vi "YKMW100 VF0 Relay Status.vi"(0 "VISA session":refnum<visa-resource-name>="MW100", 2 "Semiphore":T1, 5 "Channel_Enum":T2=1 items=["4-20_OUT", "Pres_HI1", "Pres_HI2", "Pres_LOW", "Pres_PIN", "HEATER_TOP", "HEATER_BOT", "T_Shell", "FLOWMETER", "WATT_SENSE", "WH_TICK", "Tc_1", "Tc_2", "Tc_3", "Tc_4", "Tc_5", "Tc_6", "Tc_down", "T_Shell_2", "T_Shell_3", "T_Shell_4", "RTD_IN", "RTD_OUT", "RTD_AMB", "INTF_TEMPFLO", "INTF_READY", "INTF_START", "INTF_STOP", "DRM_LOW", "DRM_HIGH", "PWR_MAIN", "VLV_DUMP", "VLV_OUT", "VLV_IN", "WATT_HOURS", "FLOW(SAMPLE)", "GALLONS", "FLOW(GPM)", "FLOW_CALC_GAIN", "FLOW_CALC_OFFSET", "FLOW_CALC_THRESHOLD", "VLV_DUMP_2", "VLV_OUT_2", "VLV_IN_2", "VLV_DUMP_3", "VLV_OUT_3", "VLV_IN_3", "VLV_DUMP_4", "VLV_OUT_4", "VLV_IN_4", "CHAN_34", "CHAN_35", "CHAN_36"], 9 "Timeout (25000)":u32=1000, 11 "error in (no error)":errorcluster) -> (4 "dup VISA session":refnum<visa-resource-name>, 6 "Output On":bool, 8 "DO Card in Slot 5":bool, 15 "error out":errorcluster)   [LabVIEW 2009]
doc: "This VI sends the message. Then it returns the response."
uses:
  ChannelSettings.ctl
panel:
  out "element":string
  out "Numeric":i32
  out "Local?":bool
  out "Read Array":string[](array[string])
  out "ENCRLF":string
  out "EACRLF":string
  # "POWER:TRUE = OFF"
  # "FALSE = CONTACT CLOSED"
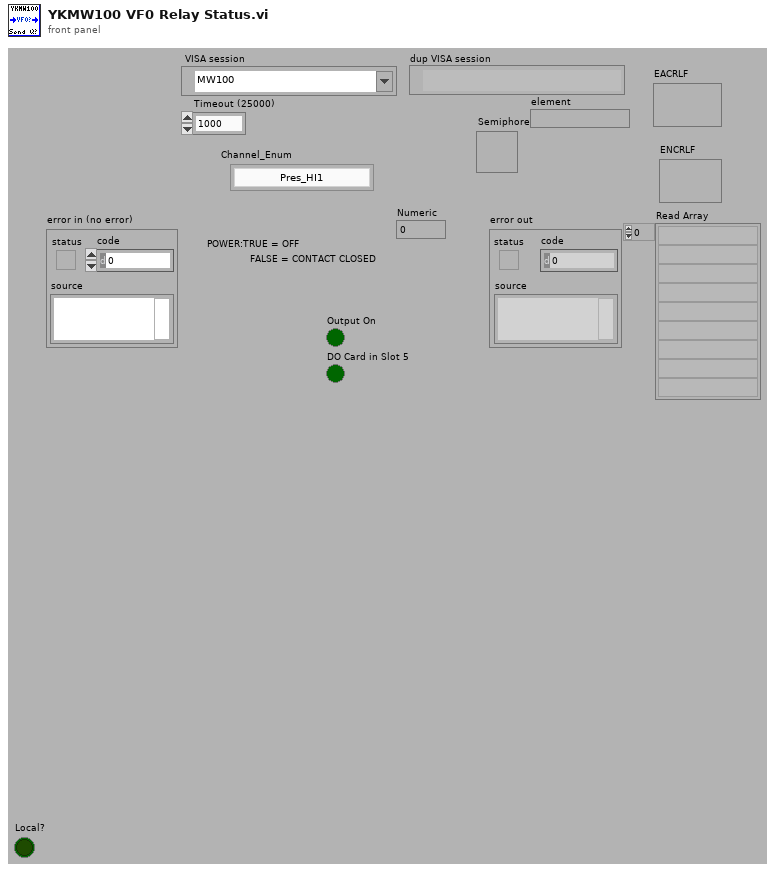
[diagram p1: front panel]
types:
  T1 = typedef "Semaphore RefNum" = refnum<k1>
  T2 = typedef "ChannelSettings.ctl" = u32
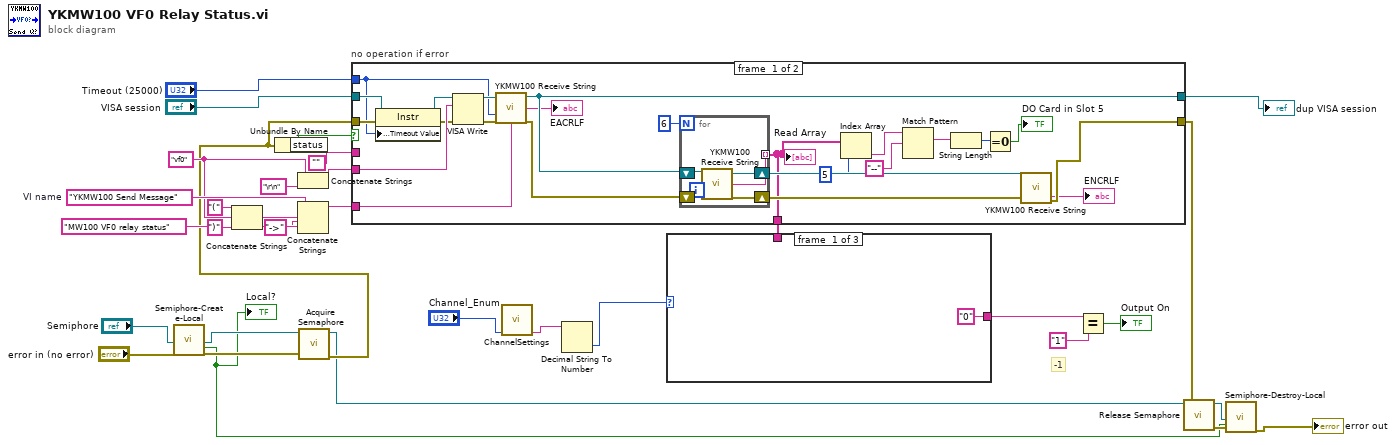
[diagram p0: block diagram]
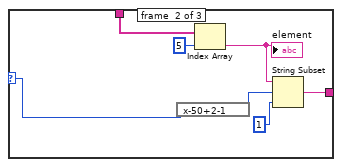
[diagram p2: hidden frame]
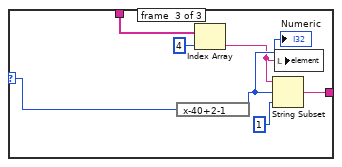
[diagram p3: hidden frame]
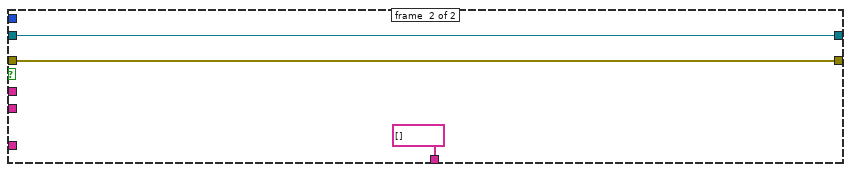
[diagram p4: hidden frame]
diagram:
  w20 = "vf0" ("Send Message (\"\")")
  w23 = "YKMW100 Send Message"  # VI name
  # "-1"
  n1 = call "Semiphore-Create-Local.vi"("Semiphore"="Semiphore", "error in (no error)"="error in (no error)") -> ("semaphore"=w13:T1, "Local?"=w6:bool, "error out"=w14:errorcluster)  [unwired: 15 in]
  "Local?" <- w6
  n2 = Concatenate Strings("(", w20, ")") -> (w24:string)
  n3 = Concatenate Strings(w20, "\r\n") -> (w33:string)
  n4 = Concatenate Strings(w23, w24, "->", "MW100 VF0 relay status" ("Source (\"\")")) -> (w29:string)
  n5 = call <vilib>:"Acquire Semaphore.vi"("error in (no error)"=w14, "semaphore"=w13) -> ("error out"=w8:errorcluster, "semaphore out"=w4:T1)  [unwired: 3 in, 1 out]
  n6 = Unbundle By Name(w8) -> ("status"=w30:bool)
  n7 = case "no operation if error" shown="False" w30 {
    tunnel: "VISA session" -> [w54 w65]
    tunnel: w33 -> [w57 _]
    tunnel: [w46 w65] -> w22
    tunnel: [w44 w64] -> w7
    tunnel: w8 -> [w56 w64]
    tunnel: w29 -> [w50 _]
    tunnel: "Timeout (25000)" -> [w49 _]
    tunnel: "" -> [_ _]
    tunnel: [w40 string[] []] -> w18
    frame #0 {
      n8 = property class="Instr"(reference=w54, error in=w56, "General Settings:Timeout Value"=w49) -> (reference out=w53:refnum<visa-resource-name>, error out=w55:errorcluster)
      n9 = VISA Write(VISA resource name=w53, write buffer=w57, error in (no error)=w55) -> (VISA resource name out=w52:refnum<visa-resource-name>, error out=w51:errorcluster)  [unwired: 1 out]
      n10 = call "YKMW100 Receive String.vi"("VISA session"=w52, "Timeout (25000)"=w49, "error in (no error)"=w51, "Source (\"\")"=w50) -> ("dup VISA session"=w46:refnum<visa-resource-name>, "Read Buffer"=→"EACRLF":string, "error out"=w45:errorcluster)  [unwired: 9 in]
      n11 = for {
        N: 6 -> [_]
        tunnel: [w58] -> w40 mode=indexing
        shift-right: [w62] -> w48
        shift-left: w46 -> [w60]
        shift-right: [w61] -> w47
        shift-left: w45 -> [w59]
        n12 = call "YKMW100 Receive String.vi"("VISA session"=w60, "error in (no error)"=w59) -> ("dup VISA session"=w62:refnum<visa-resource-name>, "Read Buffer"=w58:string, "error out"=w61:errorcluster)  [unwired: 11 in]
      }
      "Read Array" <- w40
      n13 = Index Array(array=w40, index=5) -> (element=w38:string)
      n14 = Match Pattern(string=w38, regular expression="--") -> (match substring=w36:string)  [unwired: 1 in, 3 out]
      n15 = String Length(string=w36) -> (length=w35:i32)
      n16 = Equal To 0?(x=w35) -> (x = 0?=→"DO Card in Slot 5":bool)
      n17 = call "YKMW100 Receive String.vi"("VISA session"=w48, "error in (no error)"=w47) -> ("Read Buffer"=→"ENCRLF":string, "error out"=w44:errorcluster)  [unwired: 11 in, 1 out]
    }
    frame #1 {
    }
  }
  "dup VISA session" <- w22
  n18 = call "ChannelSettings.vi"("Channel_Enum"="Channel_Enum") -> ("Channel String"=w3:string)  [unwired: 10 in]
  n19 = Decimal String To Number(string=w3) -> (number=w1:i32)  [unwired: 2 in, 1 out]
  n20 = case shown="51..60" w1 {
    selector: w1 -> [_ w67 w76]
    tunnel: w18 -> [_ w73 w80]
    tunnel: ["0" ("Read Buffer") w68 w77] -> w17
    frame #0 {
    }
    frame #1 {
      n21 = expression code="x-50+2-1"(w67) -> (w70:i32)
      n22 = Index Array(array=w73, index=5) -> (element=w71:string)
      "element" <- w71
      n23 = String Subset(string=w71, offset (0)=w70, length (rest)=1 ("length (rest)")) -> (substring=w68:string)
    }
    frame #2 {
      n24 = expression code="x-40+2-1"(w76) -> (w75:i32)
      "Numeric" <- w75
      n25 = Index Array(array=w80, index=4) -> (element=w74:string)
      n26 = String Subset(string=w74, offset (0)=w75, length (rest)=1 ("length (rest)")) -> (substring=w77:string)
      n27 = local write "element"(w74) -> ()
    }
  }
  n28 = Equal?(x=w17, y="1") -> (x = y?=→"Output On":bool)
  n29 = call <vilib>:"Release Semaphore.vi"("error in (no error)"=w7, "semaphore"=w4) -> ("error out"=w12:errorcluster, "semaphore out"=w11:T1)  [unwired: 4 in]
  n30 = call "Semiphore-Destroy-Local.vi"("Semiphore"=w11, "Local?"=w6, "error in (no error)"=w12) -> ("error out"=→"error out":errorcluster)  [unwired: 16 in]
